vi "X-Y-Z-Move_Api.vi"(5 "加速度":dbl=800.0, 7 "最高速":dbl=1150.0, 8 "Error In":errorcluster, 11 "X-Y-Z移動":dbl[](array[numeric])=[0.0, 0.0, 0.0]) -> (0 "Error Out":errorcluster, 4 "三角形?":bool)   [LabVIEW 2019]
uses:
  <vilib>/Platform/TimedLoop/XDataNode/timing_clust.ctl
  <vilib>/Platform/TimedLoop/XDataNode/nitl_modes.ctl
  <vilib>/Platform/TimedLoop/XDataNode/wakeup.ctl
  <vilib>/Platform/TimedLoop/XDataNode/XDataNode.xnode
  <vilib>/Platform/TimedLoop/XDataNode/XDNodeRunTimeDep.lvlib
panel:
  out "Waveform Chart 2":dbl(graph)
  out "Waveform Chart":dbl(graph)
  in  "Stop":bool
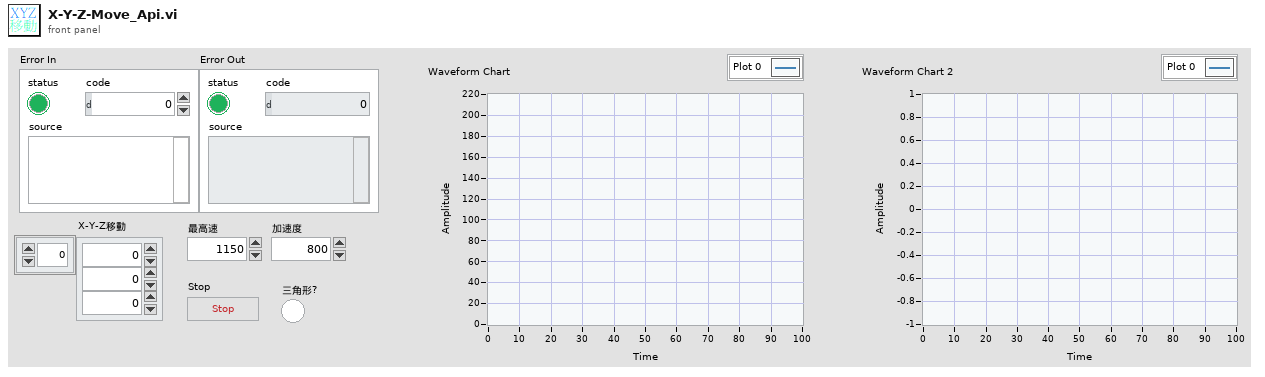
[diagram p1: front panel]
types:
  T1 = typedef "XDNodeRunTimeDep.lvlib/timing_clust.ctl" = cluster{"Expected End [f-1]":u64, "Actual End [f-1]":u64, "Finished Late? [f-1]":bool, "Expected End [i-1]":u64, "Actual End [i-1]":u64, "Finished Late? [i-1]":bool, "Expected Start [i]":u64, "Actual Start [i]":u64, "Expected Start [f]":u64, "Actual Start [f]":u64, "Source Name":string, "Structure Name":string, "Period":i64, "Deadline":i64, "Offset":i64, "Start":i64, "Priority":i32, "Timeout":i32, "Mode":T2, "Wakeup Reason":T3, "Error":errorcluster, "Source Type":string, "Secondary Source Type":string, "Global End Time":u64, "Global Start Time":u64, "Frame Duration":u64, "Iteration Duration":u64, "Assigned CPU":i32, "I/O Scan Engine Mode":u32}
  T2 = typedef "XDNodeRunTimeDep.lvlib/nitl_modes.ctl" = enum32{"No Change", "Process missed periods, maintain original phase", "Discard missed periods, maintain original phase", "Process missed periods, ignore original phase", "Discard missed periods, ignore original phase"}
  T3 = typedef "XDNodeRunTimeDep.lvlib/wakeup.ctl" = enum32{"Normal", "Aborted", "Asynchronous wakeup", "Timing source error", "Timed loop error", "Timeout"}
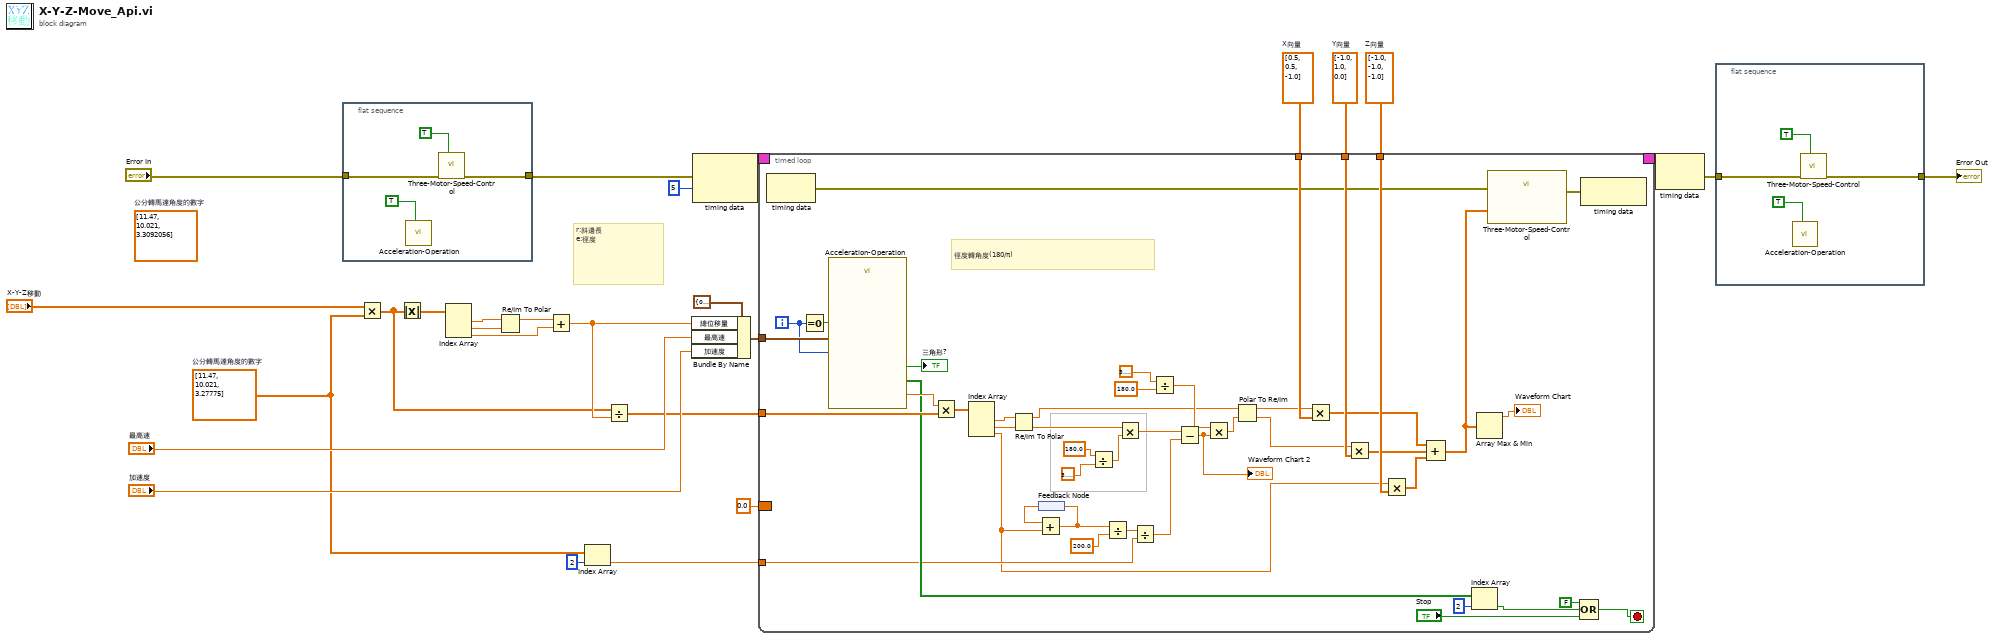
[diagram p0: block diagram]
diagram:
  (unwired) dbl[] [11.47, 10.021, 3.3092056]  # 公分轉馬達角度的數字
  w7 = dbl[] [-1.0, -1.0, -1.0]  # Z向量
  w8 = dbl[] [-1.0, 1.0, 0.0]  # Y向量
  w9 = dbl[] [0.5, 0.5, -1.0]  # X向量
  w6 = dbl[] [11.47, 10.021, 3.27775]  # 公分轉馬達角度的數字
  # "r:斜邊長\ne:徑度"
  n1 = flat-sequence {
    tunnel: "Error In" -> [w30]
    tunnel: [w29] -> w11
    frame #0 {
      n2 = call "Acceleration-Operation.vi"("Reset"=TRUE) -> ()  [unwired: 8 in, 3 out]
      n3 = call "Three-Motor-Speed-Control.vi"("Reset"=TRUE, "Error In"=w30) -> ("Error Out"=w29:errorcluster)  [unwired: 9 in]
    }
  }
  n4 = Multiply(x="X-Y-Z移動", y=w6) -> (x*y=w12:dbl[])
  n5 = Absolute Value(x=w12) -> (abs(x)=w24:dbl[])
  n6 = Index Array(array=w24) -> (element #1=w20:dbl, element #2=w25:dbl, element #3=w21:dbl)  [unwired: 3 in]
  n7 = Re/Im To Polar(2:w25, 3:w20) -> (1:w22:dbl)  [unwired: 1 out]
  n8 = Add(x=w22, y=w21) -> (x+y=w13:dbl)
  n9 = Index Array(array=w6, index=2) -> (element=w5:dbl)
  n10 = Divide(x=w12, y=w13) -> (x/y=w14:dbl[])
  n11 = Bundle By Name(cluster=cluster{"總位移量":dbl, "最高速":dbl, "加速度":dbl} {"總位移量"=0.0, "最高速"=0.0, "加速度"=0.0} ("計算設置"), "總位移量"=w13, "最高速"="最高速", "加速度"="加速度") -> (w15:cluster{"總位移量":dbl, "最高速":dbl, "加速度":dbl})
  n12 = node-c288(w11, i64 5 ("Period")) -> (w27:T1)
  n13 = timed-loop "Timed Loop" {
    timing: w27 -> [_]
    timing-out: [_] -> w26
    tunnel: w15 -> [w76]
    tunnel: w14 -> [w74]
    border: 0.0 -> [_]
    tunnel: w9 -> [w51]
    tunnel: w8 -> [w50]
    tunnel: w7 -> [w49]
    tunnel: w5 -> [w41]
    i -> [w72]
    stop <- w70 stop-if-true
    # "徑度轉角度(180/π)"
    n14 = node-c288() -> (w44:errorcluster)  [unwired: 1 in]
    n15 = Equal To 0?(x=w72) -> (x = 0?=w73:bool)
    n16 = call "Acceleration-Operation.vi"("Reset"=w73, "迴圈( I )"=w72, "計算設置"=w76) -> ("完成?"=w69:bool[], "速度"=w75:dbl, "三角形?"=→"三角形?":bool)  [unwired: 6 in]
    n17 = Multiply(x=w75, y=w74) -> (x*y=w66:dbl[])
    n18 = Index Array(array=w66) -> (element #1=w65:dbl, element #2=w64:dbl, element #3=w38:dbl)  [unwired: 3 in]
    n19 = Re/Im To Polar(2:w64, 3:w65) -> (0:w63:dbl, 1:w52:dbl)
    n20 = feedback #1() -> (w59:dbl)
    n21 = Add(x=w59, y=w38) -> (x+y=w58:dbl)
    n22 = feedback-in #1(w58) -> ()
    n23 = Divide(x=180.0, y=3.141592653589793) -> (x/y=w60:dbl)
    n24 = Divide(x=w58, y=200.0) -> (x/y=w43:dbl)
    n25 = Multiply(x=w63, y=w60) -> (x*y=w56:dbl)
    n26 = Divide(x=w43, y=w41) -> (x/y=w42:dbl)
    n27 = Divide(x=3.141592653589793, y=180.0 ("x")) -> (x/y=w53:dbl)
    n28 = Subtract(x=w56, y=w42) -> (x-y=w33:dbl)
    "Waveform Chart 2" <- w33
    n29 = Multiply(x=w53, y=w33) -> (x*y=w35:dbl)
    n30 = Polar To Re/Im(2:w35, 3:w52) -> (0:w36:dbl, 1:w37:dbl)
    n31 = Multiply(x=w37, y=w51) -> (x*y=w48:dbl[])
    n32 = Multiply(x=w36, y=w50) -> (x*y=w47:dbl[])
    n33 = Multiply(x=w38, y=w49) -> (x*y=w46:dbl[])
    n34 = Compound Arithmetic op=ADD(w48, w47, w46) -> (w32:dbl[])
    n35 = Index Array(array=w69, index=2) -> (element=w40:bool)
    n36 = Array Max & Min(array=w32) -> (max value=→"Waveform Chart":dbl)  [unwired: 3 out]
    n37 = call "Three-Motor-Speed-Control.vi"("Error In"=w44, "速度(秒/度)"=w32) -> ("Error Out"=w45:errorcluster)  [unwired: 9 in]
    n38 = Compound Arithmetic op=OR(FALSE ("value"), w40, "Stop") -> (w70:bool)
    n39 = node-c288(w45) -> ()  [unwired: 1 out]
  }
  n40 = node-c288(w26) -> (w3:errorcluster)
  n41 = flat-sequence {
    tunnel: [w85] -> w2
    tunnel: w3 -> [w82]
    frame #0 {
      n42 = call "Acceleration-Operation.vi"("Reset"=TRUE) -> ()  [unwired: 8 in, 3 out]
      n43 = call "Three-Motor-Speed-Control.vi"("Reset"=TRUE, "Error In"=w82) -> ("Error Out"=w85:errorcluster)  [unwired: 9 in]
    }
  }
  "Error Out" <- w2
